vi "Write.vi"(8 "error in (no error)":errorcluster, 9 "timeout (ms)":i32=1000, 10 "CAN Data":T1[](array[typedef]) {"Tags" format="%.0x"; "payload" format="%x"; "identifier" format="%x"}, 11 "CAN_Logic in":refnum<class "CAN_Logic.lvclass">) -> (0 "error out":errorcluster, 3 "CAN_Logic out":refnum<class "CAN_Logic.lvclass">)   [LabVIEW 2021, in "CAN_Logic.lvclass"]
uses:
  CAN_Logic.lvclass
  Channels/ChannelRegistrar/typedef/Datatype CAN.ctl
  CAN_Logic.lvclass/CAN_Logic.ctl
  <vilib>/xnet/xnet.llb/XNET Frame CAN.ctl
  <vilib>/xnet/xnet.llb/XNET Frame Type CAN.ctl
  <vilib>/xnet/xnet.llb/XNET Write (Frame CAN).vi
  Channels/ChannelRegistrar/ChannelRegistrar.lvlib
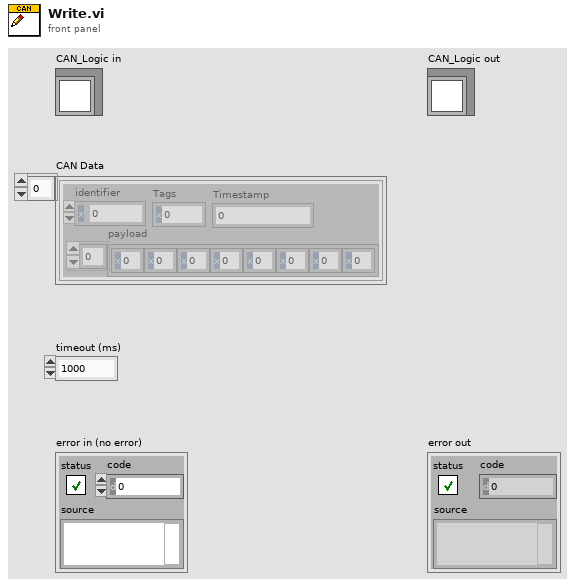
[diagram p1: front panel]
types:
  T1 = typedef "ChannelRegistrar.lvlib/Datatype CAN.ctl" = cluster{"payload":u8[], "identifier":u32, "Tags":u8, "Timestamp":u64}
  T2 = typedef "XNET Frame CAN.ctl" = cluster{"timestamp":timestamp, "payload":u8[], "identifier":u32, "type":T3, "extended?":bool, "echo?":bool}
  T3 = typedef "XNET Frame Type CAN.ctl" = u8
  T4 = typedef "CAN_Logic.lvclass/ISO FD Frame Type.ctl" = enum16{"Not Specified", "CAN 2.0", "FD", "FD+BRS"}
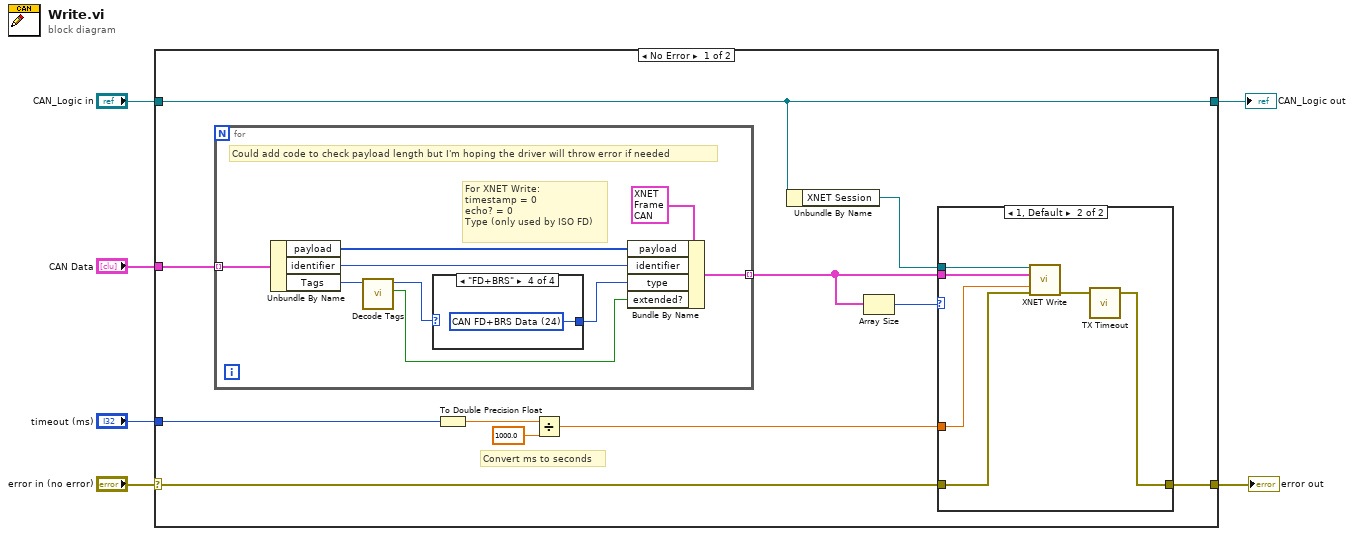
[diagram p0: block diagram]
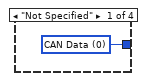
[diagram p3: hidden frame]
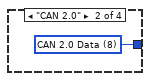
[diagram p4: hidden frame]
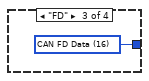
[diagram p5: hidden frame]
diagram:
  n1 = case shown="No Error" "error in (no error)" {
    selector: "error in (no error)" -> [w15 w39]
    tunnel: [w14 w39] -> w5
    tunnel: [w17 w38] -> w3
    tunnel: "CAN_Logic in" -> [w17 w38]
    tunnel: "CAN Data" -> [w13 _]
    tunnel: "timeout (ms)" -> [w8 _]
    frame No Error {
      # "Convert ms to seconds"
      n2 = for {
        tunnel: w13 -> [w33] mode=indexing
        tunnel: [w31] -> w12 mode=indexing
        # "Could add code to check payload length but I'm hoping the driver will throw error if needed"
        # "For XNET Write:\ntimestamp = 0\necho? = 0\nType (only used by ISO FD)"
        n3 = Unbundle By Name(w33) -> ("payload"=w29:u8[], "identifier"=w28:u32, "Tags"=w27:u8)
        n4 = call "Decode Tags.vi"("Tags in"=w27) -> ("Extended ID"=w25:bool, "ISO FD Type"=w26:T4)  [unwired: 8 in, 1 out]
        n5 = case shown="\"FD+BRS\"" w26 {
          tunnel: [w34 w35 w36 w37] -> w30
          frame "Not Specified" {
            w34 = T3 0 items=["CAN Data"=0, "CAN Remote"=1, "CAN Bus Error"=2, "CAN 2.0 Data"=8, "CAN FD Data"=16, "CAN FD+BRS Data"=24, "J1939 Data"=192, "Delay"=224, "Log Trigger"=225, "Start Trigger"=226] ("type")
          }
          frame "CAN 2.0" {
            w35 = T3 8 items=["CAN Data"=0, "CAN Remote"=1, "CAN Bus Error"=2, "CAN 2.0 Data"=8, "CAN FD Data"=16, "CAN FD+BRS Data"=24, "J1939 Data"=192, "Delay"=224, "Log Trigger"=225, "Start Trigger"=226] ("type")
          }
          frame "FD" {
            w36 = T3 16 items=["CAN Data"=0, "CAN Remote"=1, "CAN Bus Error"=2, "CAN 2.0 Data"=8, "CAN FD Data"=16, "CAN FD+BRS Data"=24, "J1939 Data"=192, "Delay"=224, "Log Trigger"=225, "Start Trigger"=226] ("type")
          }
          frame "FD+BRS" {
            w37 = T3 24 items=["CAN Data"=0, "CAN Remote"=1, "CAN Bus Error"=2, "CAN 2.0 Data"=8, "CAN FD Data"=16, "CAN FD+BRS Data"=24, "J1939 Data"=192, "Delay"=224, "Log Trigger"=225, "Start Trigger"=226] ("type")
          }
        }
        n6 = Bundle By Name(cluster=T2 {"timestamp"=timestamp(0 s since 1904-01-01), "payload"=[], "identifier"=0, "type"=0, "extended?"=FALSE, "echo?"=FALSE} ("CAN frame"), "payload"=w29, "identifier"=w28, "type"=w30, "extended?"=w25) -> (w31:T2)
      }
      n7 = To Double Precision Float(number=w8) -> (double precision float=w10:dbl)
      n8 = Divide(x=w10, y=1000.0) -> (x/y=w7:dbl)
      n9 = Unbundle By Name(w17) -> ("XNET Session"=w16:refnum<k21>)
      n10 = Array Size(array=w12) -> (size(s)=w11:i32)
      n11 = case shown="1, Default" w11 {
        tunnel: w16 -> [_ w24]
        tunnel: w15 -> [w18 w23]
        tunnel: [w18 w19] -> w14
        tunnel: w12 -> [_ w22]
        tunnel: w7 -> [_ w21]
        frame 0 {
        }
        frame 1, Default {
          n12 = call-poly <vilib>:"XNET Write.vi"("session in"=w24, "data"=w22, "timeout (10)"=w21, "error in (no error)"=w23) -> ("error out"=w20:errorcluster)  [unwired: 10 in, 1 out]
          n13 = call "TX Timeout.vi"("error in (no error)"=w20) -> ("error out"=w19:errorcluster)  [unwired: 3 in]
        }
      }
    }
    frame Error {
    }
  }
  "error out" <- w5
  "CAN_Logic out" <- w3
